vi "Update RPC Method Template.vi"(8 "error in (no error)":errorcluster, 11 "Server Library (Library Item) in":refnum<vi>) -> (0 "error out":errorcluster, 3 "Server Library (Library Item) out":refnum<vi>)   [LabVIEW 2019, in "gRPC Scripting Tools.lvlib"]
uses:
  gRPC Scripting Tools.lvlib
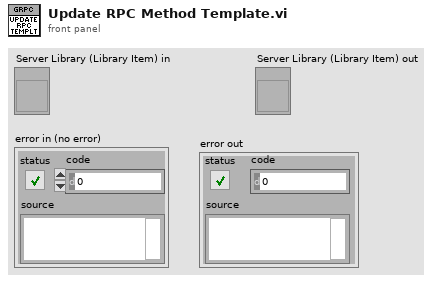
[diagram p1: front panel]
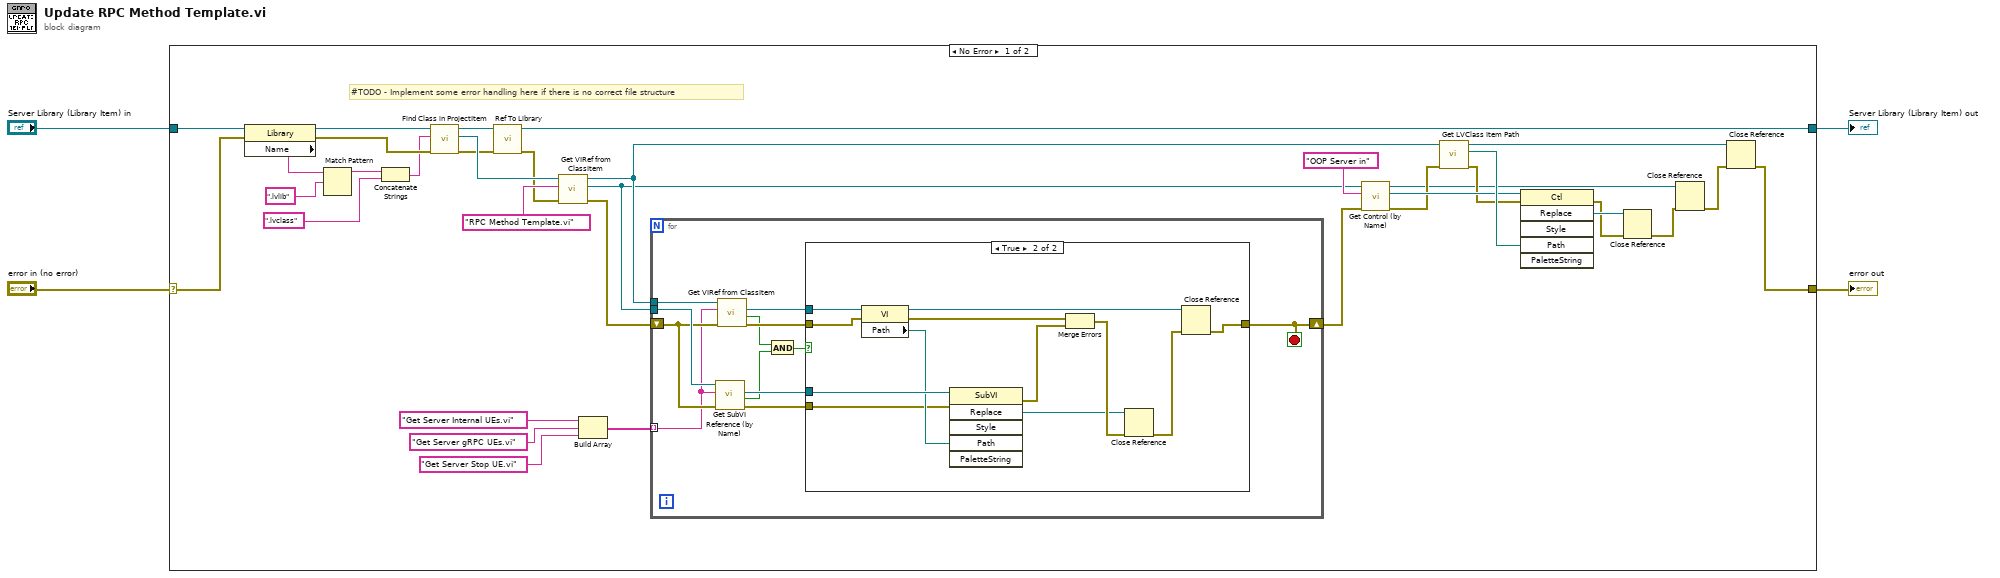
[diagram p0: block diagram]
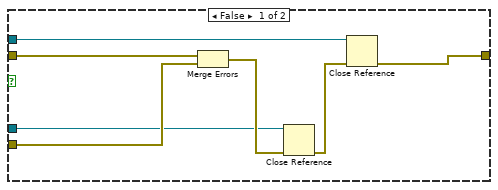
[diagram p2: hidden frame]
diagram:
  n1 = case shown="No Error" "error in (no error)" {
    selector: "error in (no error)" -> [w9 w72]
    tunnel: "Server Library (Library Item) in" -> [w27 w71]
    tunnel: [w10 w72] -> w3
    tunnel: [w7 w71] -> w1
    frame No Error {
      # "#TODO - Implement some error handling here if there is no correct file structure"
      n2 = property class="Library"(reference=w27, error in=w9) -> (reference out=w24:refnum<vi>, error out=w26:errorcluster, "Name"=w20:string)
      n3 = Match Pattern(string=w20, regular expression=".lvlib") -> (before substring=w22:string)  [unwired: 1 in, 3 out]
      n4 = Concatenate Strings(w22, ".lvclass" ("string")) -> (w25:string)
      n5 = call "Find Class in ProjectItem.vi"("error in (no error)"=w26, "Class Name"=w25, "ProjectItem in"=w24) -> ("error out"=w6:errorcluster, "LVClass out"=w29:refnum<vi>, "ProjectItem out"=w8:refnum<vi>)  [unwired: 5 in, 1 out]
      n6 = call "Ref To Library.vi"("error in (no error)"=w6, "ProjectItem in"=w8) -> ("error out"=w5:errorcluster, "Library out"=w7:refnum<vi>)  [unwired: 8 in]
      n7 = call "Get VIRef from ClassItem.vi"("error in (no error)"=w5, "Item Name"="RPC Method Template.vi", "LVClassLibrary in"=w29) -> ("error out"=w30:errorcluster, "VIref out"=w35:refnum<vi>, "LVClassLibrary out"=w38:refnum<vi>)  [unwired: 5 in, 1 out]
      n8 = Build Array("Get Server Internal UEs.vi" ("SubVI Name"), "Get Server gRPC UEs.vi" ("SubVI Name"), "Get Server Stop UE.vi" ("SubVI Name")) -> (w34:string[])
      n9 = for {
        tunnel: w35 -> [w51]
        tunnel: w34 -> [w45] mode=indexing
        shift-right: [w40] -> w18
        shift-left: w30 -> [w49]
        tunnel: w38 -> [w41]
        stop <- w40 stop-if-true
        n10 = call "Get SubVI Reference (by Name).vi"("error in (no error)"=w49, "SubVI Name"=w45, "Owner VI in"=w51) -> ("error out"=w46:errorcluster, "Found ?"=w43:bool, "SubVI Refnum out"=w50:refnum<vi>)  [unwired: 5 in, 1 out]
        n11 = call "Get VIRef from ClassItem.vi"("error in (no error)"=w49, "Item Name"=w45, "LVClassLibrary in"=w41) -> ("error out"=w47:errorcluster, "Found ?"=w44:bool, "VIref out"=w48:refnum<vi>)  [unwired: 5 in, 1 out]
        n12 = And(x=w44, y=w43) -> (x .and. y?=w42:bool)
        n13 = case shown="True" w42 {
          tunnel: w50 -> [w53 w70]
          tunnel: w48 -> [w57 w69]
          tunnel: w47 -> [w55 w61]
          tunnel: w46 -> [w56 w67]
          tunnel: [w52 w60] -> w40
          frame False {
            n14 = Merge Errors(w55, w56) -> (w54:errorcluster)
            n15 = Close Reference(reference=w53, error in (no error)=w54) -> (error out=w58:errorcluster)
            n16 = Close Reference(reference=w57, error in (no error)=w58) -> (error out=w52:errorcluster)
          }
          frame True {
            n17 = property class="VI"(reference=w69, error in=w61) -> (reference out=w62:refnum<vi>, error out=w65:errorcluster, "Path"=w68:path)
            n18 = invoke class="SubVI" method="Replace"(reference=w70, error in=w67, "Path"=w68) -> (error out=w66:errorcluster, "Replace"=w63:refnum<vi>)  [unwired: 3 in, 4 out]
            n19 = Merge Errors(w65, w66) -> (w64:errorcluster)
            n20 = Close Reference(reference=w63, error in (no error)=w64) -> (error out=w59:errorcluster)
            n21 = Close Reference(reference=w62, error in (no error)=w59) -> (error out=w60:errorcluster)
          }
        }
      }
      n22 = call "Get Control (by Name).vi"("error in (no error)"=w18, "Control Label"="OOP Server in" ("Constant Label"), "Owner VI in"=w35) -> ("error out"=w19:errorcluster, "Control Refnum"=w37:refnum<vi>, "Owner VI out"=w13:refnum<vi>)  [unwired: 5 in, 1 out]
      n23 = call "Get LVClass Item Path.vi"("error in (no error)"=w19, "LVClassLibrary in"=w38) -> ("error out"=w17:errorcluster, "Path"=w39:path, "LVClassLibrary out"=w12:refnum<vi>)  [unwired: 7 in]
      n24 = invoke class="Ctl" method="Replace"(reference=w37, error in=w17, "Path"=w39) -> (error out=w15:errorcluster, "Replace"=w16:refnum<vi>)  [unwired: 3 in, 4 out]
      n25 = Close Reference(reference=w16, error in (no error)=w15) -> (error out=w14:errorcluster)
      n26 = Close Reference(reference=w13, error in (no error)=w14) -> (error out=w11:errorcluster)
      n27 = Close Reference(reference=w12, error in (no error)=w11) -> (error out=w10:errorcluster)
    }
    frame Error {
    }
  }
  "error out" <- w3
  "Server Library (Library Item) out" <- w1
